vi "2 - Generate Post-Install.vi"() -> ()   [LabVIEW 2020]
uses:
  <vilib>/zip/NI_Unzip.lvlib
panel:
  out "error out":errorcluster
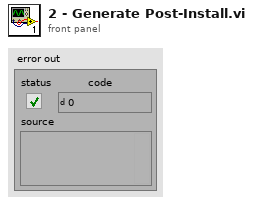
[diagram p1: front panel]
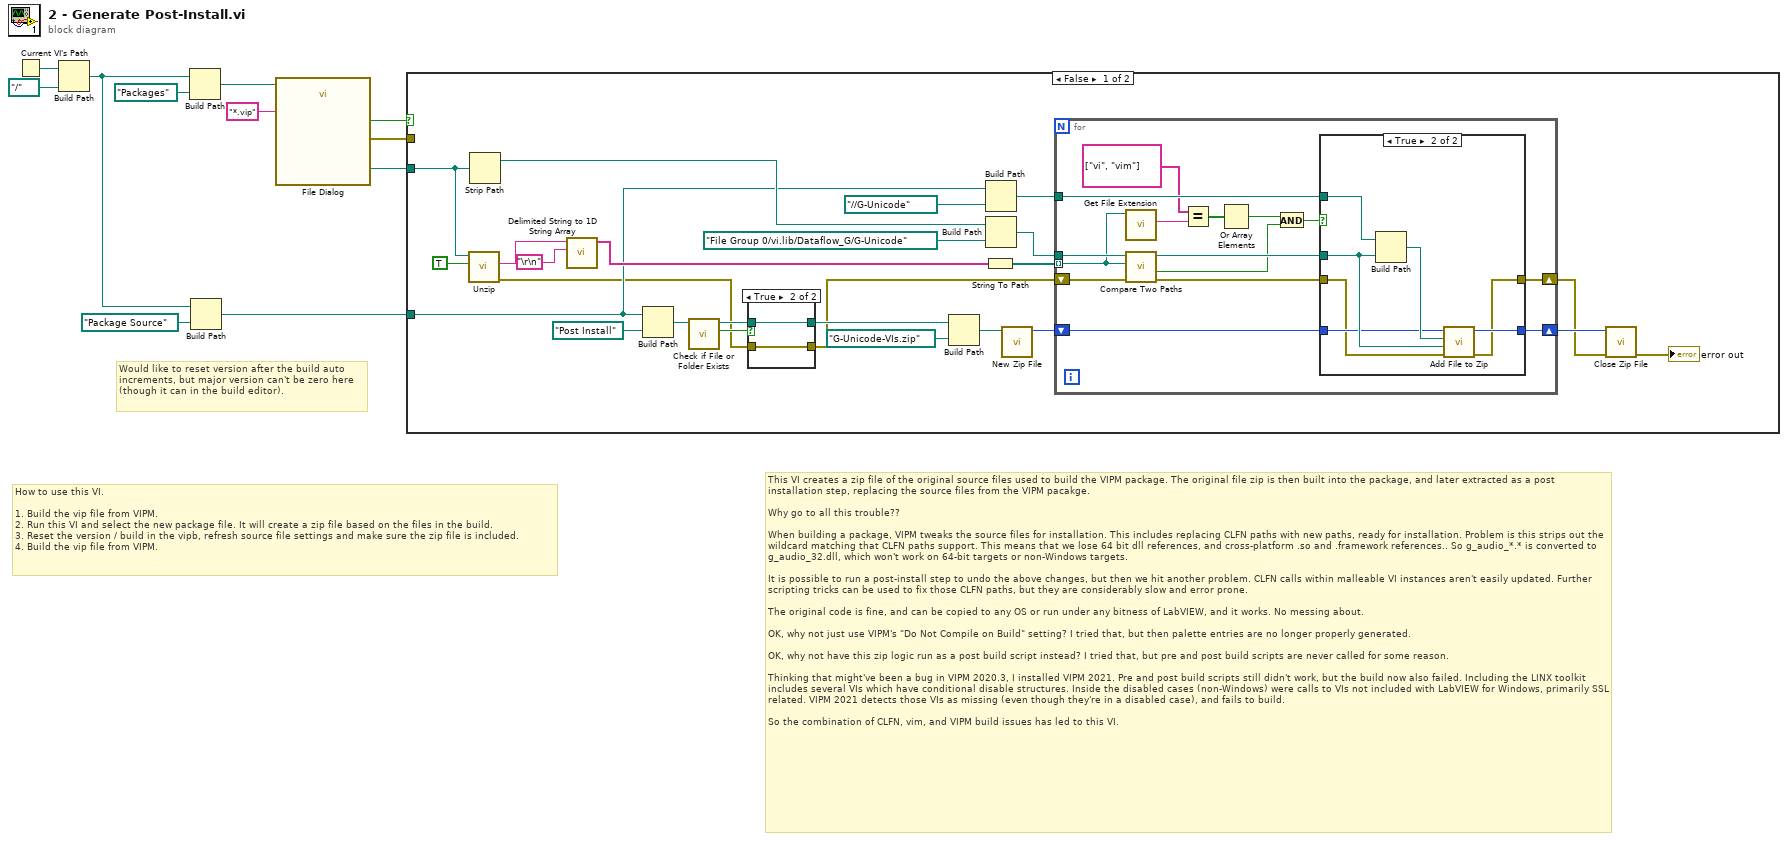
[diagram p0: block diagram]
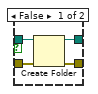
[diagram p2: hidden frame]
diagram:
  # "Would like to reset version after the build auto increments, but major version can't be zero here (though it can in the build editor)."
  # "How to use this VI.\n\n1. Build the vip file from VIPM.\n2. Run this VI and select the new package file. It will create a zip file based on the files in the build.\n3. Reset the version / build in the vipb, refresh source file settings and make sure the zip file is included.\n4. Build the vip file from VIPM."
  # "This VI creates a zip file of the original source files used to build the VIPM package. The original file zip is then built into the package, and later extracted as a post installation step, replacing the source files from the VIPM pacakge.\n\nWhy go to all this trouble??\n\nWhen building a package, VIPM tweaks the source files for installation. This includes replacing CLFN paths with new paths, ready for installation. Problem is this strips out the wildcard matching that CLFN paths support. This means that we lose 64 bit dll references, and cross-platform .so and .framework references.. So g_audio_*.* is converted to g_audio_32.dll, which won't work on 64-bit targets or non-Windows targets.\n\nIt is possible to run a post-install step to undo the above changes, but then we hit another problem. CLFN calls within malleable VI instances aren't easily updated. Further scripting tricks can be used to fix those CLFN paths, but they are considerably slow and error prone.\n\nThe original code is fine, and can be copied to any OS or run under any bitness of LabVIEW, and it works. No messing about.\n\nOK, why not just use VIPM's \"Do Not Compile on Build\" setting? I tried that, but then palette entries are no longer properly generated.\n\nOK, why not have this zip logic run as a post build script instead? I tried that, but pre and post build scripts are never called for some reason.\n\nThinking that might've been a bug in VIPM 2020.3, I installed VIPM 2021. Pre and post build scripts still didn't work, but the build now also failed. Including the LINX toolkit includes several VIs which have conditional disable structures. Inside the disabled cases (non-Windows) were calls to VIs not included with LabVIEW for Windows, primarily SSL related. VIPM 2021 detects those VIs as missing (even though they're in a disabled case), and fails to build.\n\nSo the combination of CLFN, vim, and VIPM build issues has led to this VI."
  n1 = Current VI's Path() -> (path=w7:path)
  n2 = Build Path(base path=w7, name or relative path=path "../..") -> (appended path=w2:path)
  n3 = Build Path(base path=w2, name or relative path=path "Packages") -> (appended path=w4:path)
  n4 = Build Path(base path=w2, name or relative path=path "Package Source") -> (appended path=w1:path)
  n5 = call "File Dialog"("start path"=w4, "pattern (all files)"="*.vip") -> ("selected path"=w8:path, "cancelled"=w11:bool, "error out"=w10:errorcluster)  [unwired: 10 in, 1 out]
  n6 = case shown="False" w11 {
    tunnel: w1 -> [w18 _]
    tunnel: w10 -> [_ _]
    tunnel: w8 -> [w25 _]
    frame False {
      n7 = call <vilib>:"Unzip.vi"("Preview only?"=TRUE, "Zip file"=w25) -> ("error out"=w13:errorcluster, "Preview"=w22:string)  [unwired: 7 in, 1 out]
      n8 = Strip Path(path=w25) -> (stripped path=w24:path)  [unwired: 1 out]
      n9 = call <vilib>:"Delimited String to 1D String Array.vi"("delimiter"="\r\n", "delimited string"=w22) -> ("string array"=w20:string[])  [unwired: 9 in]
      n10 = Build Path(base path=w18, name or relative path=path "Post Install") -> (appended path=w16:path)
      n11 = call <vilib>:"Check if File or Folder Exists.vi"("path"=w16) -> ("file or folder exists?"=w14:bool, "dup path"=w15:path)  [unwired: 8 in, 1 out]
      n12 = case shown="True" w14 {
        tunnel: [w40 w42] -> w17
        tunnel: w15 -> [w39 w42]
        tunnel: w13 -> [w38 w41]
        tunnel: [w37 w41] -> w12
        frame False {
          n13 = Create Folder(path (use dialog)=w39, error in=w38) -> (created path=w40:path, error out=w37:errorcluster)  [unwired: 1 in, 1 out]
        }
        frame True {
        }
      }
      n14 = Build Path(base path=w17, name or relative path=path "G-Unicode-VIs.zip") -> (appended path=w31:path)
      n15 = String To Path(string=w20) -> (path=w26:path[])
      n16 = Build Path(base path=w18, name or relative path=path "../../G-Unicode") -> (appended path=w33:path)
      n17 = Build Path(base path=w24, name or relative path=path "File Group 0/vi.lib/Dataflow_G/G-Unicode") -> (appended path=w35:path)
      n18 = call <vilib>:"New Zip File.vi"("target"=w31) -> ("zip file out"=w30:i64)  [unwired: 4 in, 2 out]
      n19 = for {
        tunnel: w35 -> [w44]
        tunnel: w26 -> [w43] mode=indexing
        tunnel: w33 -> [w51]
        shift-right: [w54] -> w28
        shift-left: w12 -> [w56]
        shift-right: [w52] -> w29
        shift-left: w30 -> [w53]
        n20 = call <vilib>:"Get File Extension.vi"("file"=w43) -> ("lowercase file extension"=w50:string)  [unwired: 6 in, 4 out]
        n21 = call <vilib>:"Compare Two Paths.vi"("error in (no error)"=w56, "Path 2"=w43, "Path 1"=w44) -> ("error out"=w55:errorcluster, "Path 2 Relative to Path 1?"=w48:bool, "Relative Path from 1 to 2"=w57:path)  [unwired: 5 in, 1 out]
        n22 = Equal?(x=string[] ["vi", "vim"], y=w50) -> (x = y?=w47:bool[])
        n23 = Or Array Elements(Boolean array=w47) -> (logical OR=w46:bool)
        n24 = And(x=w46, y=w48) -> (x .and. y?=w45:bool)
        n25 = case shown="True" w45 {
          tunnel: w57 -> [_ w64]
          tunnel: w51 -> [_ w66]
          tunnel: w55 -> [w59 w61]
          tunnel: [w59 w60] -> w54
          tunnel: w53 -> [w58 w63]
          tunnel: [w58 w62] -> w52
          frame False {
          }
          frame True {
            n26 = Build Path(base path=w66, name or relative path=w64) -> (appended path=w65:path)
            n27 = call <vilib>:"Add File to Zip.vi"("error in (no error)"=w61, "destination path in zip"=w64, "source file path"=w65, "zip file in"=w63) -> ("error out"=w60:errorcluster, "zip file out"=w62:i64)  [unwired: 6 in]
          }
        }
      }
      n28 = call <vilib>:"Close Zip File.vi"("error in (no error)"=w28, "zip file in"=w29) -> ("error out"=→"error out":errorcluster)  [unwired: 5 in]
    }
    frame True {
    }
  }
